vi "Read Digital Inputs Status.vi"(8 "error in (no error)":errorcluster, 11 "PXI6521 in":refnum<class "PXI6521.lvclass">) -> (0 "error out":errorcluster, 3 "PXI6521 out":refnum<class "PXI6521.lvclass">)   [LabVIEW 2018, in "PXI6521.lvlib" / "PXI6521.lvclass"]
uses:
  PXI6521.lvclass
  Custom Controls/DAQmx Lines Scope.ctl
  Custom Controls/DAQmx Digital Scope.ctl
  PXI6521.lvclass/PXI6521.ctl
  <vilib>/DAQmx/read.llb/DAQmx Read (Digital 1D Bool 1Chan 1Samp).vi
  <vilib>/DAQmx/create/channels.llb/DAQmx Create Channel (DI-Digital Input).vi
  <vilib>/DAQmx/miscellaneous.llb/DAQmx Fill In Error Info.vi
  PPLs/DigitalIO/Parent/DigitalIO.lvlibp/DigitalIO.lvclass
  C:/Projects/LabVIEW/PPLs/DigitalIO/Parent/DigitalIO.lvlibp/DigitalIO.lvclass
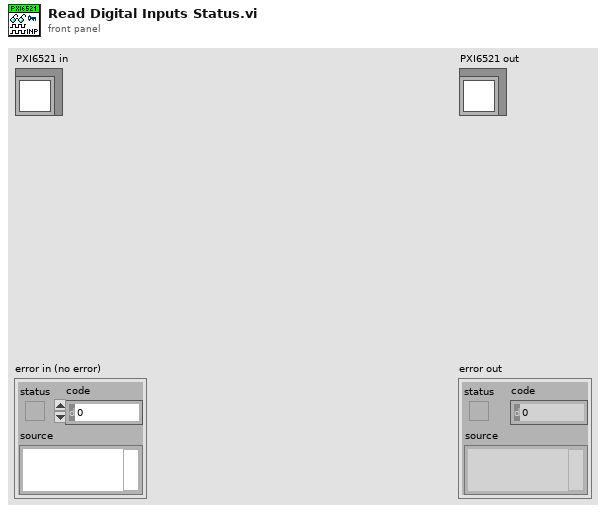
[diagram p1: front panel]
types:
  T1 = typedef "PXI6521.lvlib/PXI6521.lvclass/DAQmx Digital Scope.ctl" = enum16{"Input", "Output"}
  T2 = typedef "PXI6521.lvlib/PXI6521.lvclass/DAQmx Lines Scope.ctl" = enum16{"Full Range", "Custom Range", "Single"}
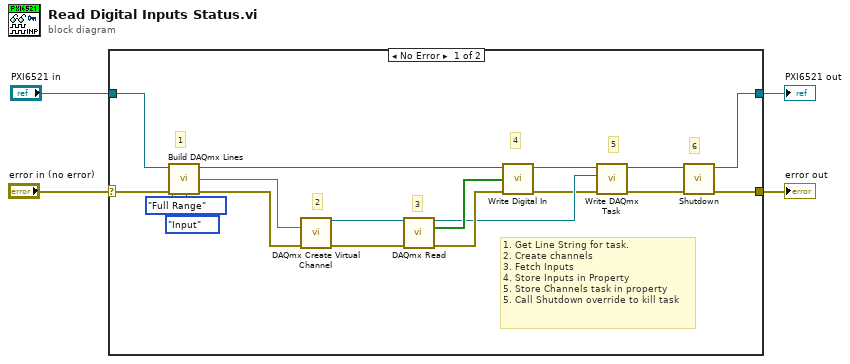
[diagram p0: block diagram]
diagram:
  n1 = case shown="No Error" "error in (no error)" {
    selector: "error in (no error)" -> [w17 w24]
    tunnel: [w5 w24] -> w3
    tunnel: [w6 w23] -> w1
    tunnel: "PXI6521 in" -> [w14 w23]
    frame No Error {
      # "6"
      # "1. Get Line String for task.\n2. Create channels\n3. Fetch Inputs\n4. Store Inputs in Property\n5. Store Channels task in property\n5. Call Shutdown override to kill task"
      # "5"
      # "4"
      # "3"
      # "2"
      # "1"
      n2 = call "Build DAQmx Lines.vi"("error in (no error)"=w17, "DAQmx Digital Scope"=DAQmx_Digital_Scope."Input", "DAQmx Lines Scope"=DAQmx_Lines_Scope."Full Range", "PXI6521 in"=w14) -> ("error out"=w12:errorcluster, "Full Line"=w20:string, "PXI6521 out"=w13:refnum<class "PXI6521.lvclass">)  [unwired: 5 in]
      n3 = call-poly <vilib>:"DAQmx Create Virtual Channel.vi"("lines"=w20, "error in"=w12) -> ("task out"=w21:refnum<k21>, "error out"=w22:errorcluster)  [unwired: 12 in]
      n4 = call-poly <vilib>:"DAQmx Read.vi"("task/channels in"=w21, "error in"=w22) -> ("task out"=w10:refnum<k21>, "data"=w15:bool[], "error out"=w16:errorcluster)  [unwired: 11 in]
      n5 = call "Write Digital In.vi"("error in (no error)"=w16, "Digital In"=w15, "DigitalIO in"=w13) -> ("error out"=w9:errorcluster, "DigitalIO out"=w11:refnum<class "PXI6521.lvclass">)  [unwired: 7 in]
      n6 = call "Write DAQmx Task.vi"("error in (no error)"=w9, "DAQmx Task"=w10, "PXI6521 in"=w11) -> ("error out"=w8:errorcluster, "PXI6521 out"=w7:refnum<class "PXI6521.lvclass">)  [unwired: 7 in]
      n7 = call "Shutdown.vi"("error in (no error)"=w8, "DigitalIO in"=w7) -> ("error out"=w5:errorcluster, "DigitalIO out"=w6:refnum<class "PXI6521.lvclass">)  [unwired: 8 in]
    }
    frame Error {
    }
  }
  "error out" <- w3
  "PXI6521 out" <- w1
